vi "Port.vi"(8 "error in (no error)":errorcluster, 11 "Node Ptr":T2 format="%.0x") -> (0 "error out":errorcluster)   [LabVIEW 2020, in "Communication Bus Template System Explorer.lvlib" / "Implementation.lvlib"]
uses:
  Implementation.lvlib
  <vilib>/NI VeriStand/Custom Device API/Custom Device Item Ref.ctl
  Types/XNET Interface Name.ctl
  <vilib>/NI VeriStand/Custom Device API/Custom Device API.lvlib
  Scripting/Communication Bus Template Scripting.lvlib
panel:
  out "CAN Cluster":string
  in  "XNET Interface Name":T1
  in  "Baud Rate":u32
  in  "Database":string(combo)
  in  "SHDocVw.IWebBrowser":refnum<k7>(container)
  in  "Specific Header":cluster{"Section Name":string}={"Section Name"="Specific Page Settings"}
  in  "General Header":cluster{"Section Name":string}={"Section Name"="General Page Settings"}
  in  "Description":string
  in  "Name":string
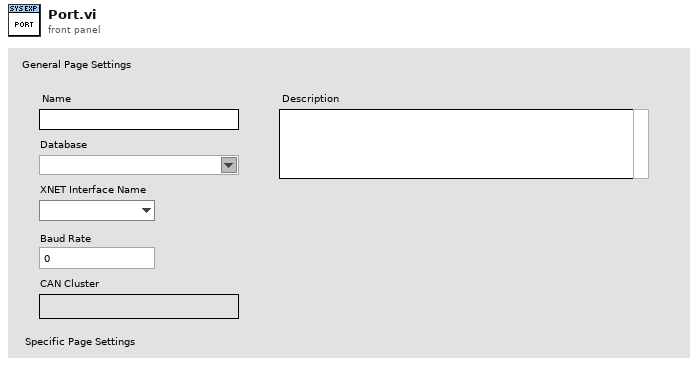
[diagram p1: front panel]
types:
  T1 = typedef "Communication Bus Template System Explorer.lvlib/Implementation.lvlib/XNET Interface Name.ctl" = u16
  T2 = typedef "Custom Device API.lvlib/Custom Device Item Ref.ctl" = u64
  T3 = typedef "Custom Device API.lvlib/Custom Device Item Info.ctl" = cluster{"Name":string, "Is Channel":bool, "GUID":string, "Is Waveform":bool}
  T4 = typedef "Custom Device API.lvlib/Custom Device Commands.ctl" = enum16{"Default", "Item renamed", "Shutdown", "Dynamic button pressed"}
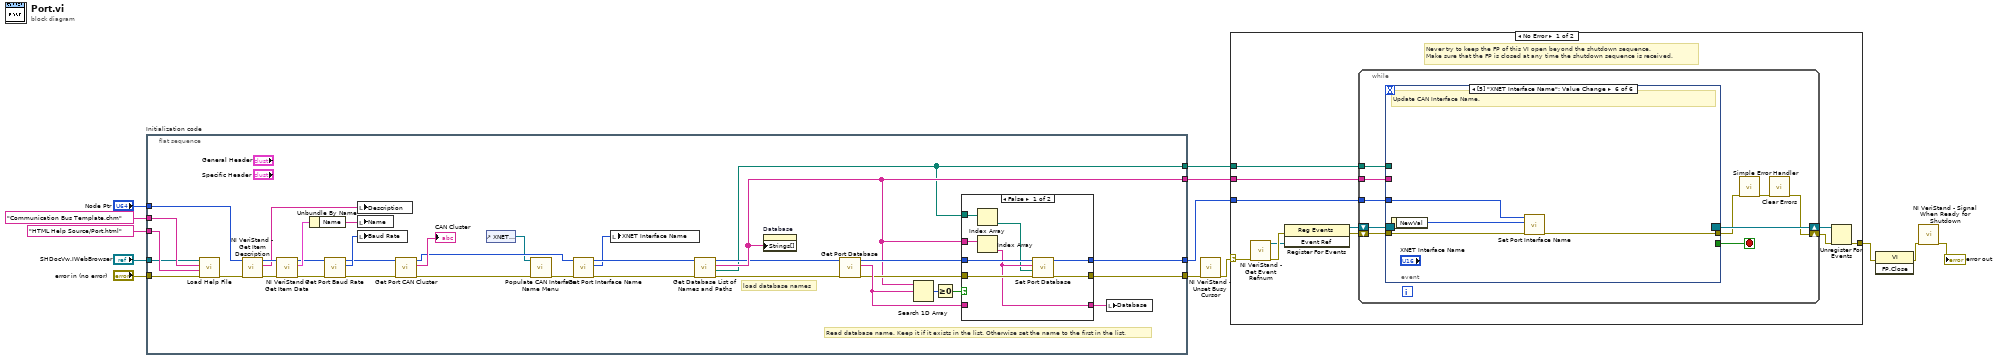
[diagram p0: block diagram]
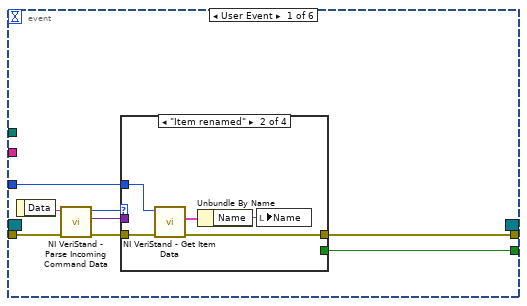
[diagram p3: hidden frame]
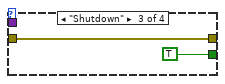
[diagram p5: hidden frame]
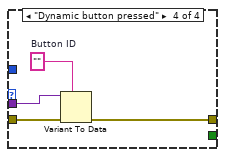
[diagram p6: hidden frame]
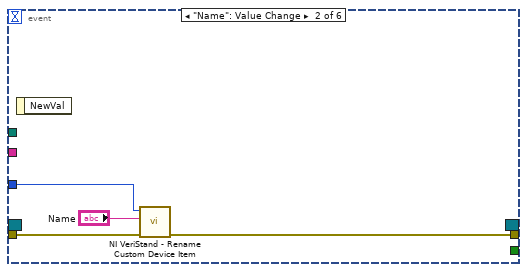
[diagram p7: hidden frame]
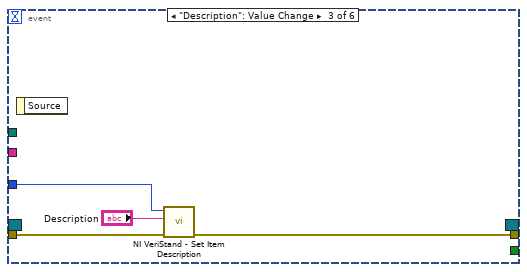
[diagram p8: hidden frame]
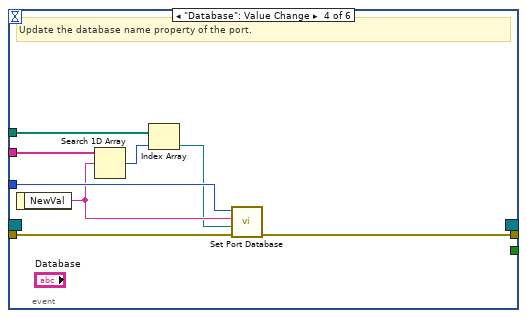
[diagram p9: hidden frame]
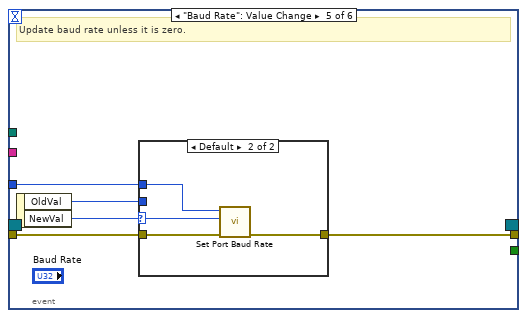
[diagram p10: hidden frame]
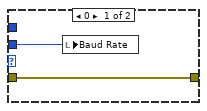
[diagram p11: hidden frame]
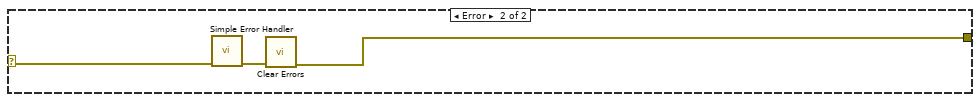
[diagram p12: hidden frame]
diagram:
  n1 = flat-sequence "Initialization code" {
    tunnel: "error in (no error)" -> [w43]
    tunnel: "Node Ptr" -> [w46]
    tunnel: [w23] -> w9
    tunnel: [w24] -> w6
    tunnel: "SHDocVw.IWebBrowser" -> [w39]
    tunnel: "HTML Help Source/Port.html" ("CD_CHM_Section") -> [w41]
    tunnel: "Communication Bus Template.chm" ("CD_CHM_FileName") -> [w40]
    tunnel: [w26] -> w2
    tunnel: [w30] -> w1
    frame #0 {
      # "Read database name. Keep it if it exists in the list. Otherwise set the name to the first in the list."
      # "load database names"
      n2 = call "Load Help File.vi"("error in (no error)"=w43, "HTML File to Load"=w41, "Main CHM File"=w40, "Browser"=w39) -> ("error out"=w42:errorcluster)  [unwired: 7 in]
      n3 = call <vilib>:"NI VeriStand - Get Item Description.vi"("error in (no error)"=w42, "Item Ref in"=w46) -> ("error out"=w48:errorcluster, "Description"=w44:string, "Item Ref out"=w49:T2)  [unwired: 7 out]
      n4 = call <vilib>:"NI VeriStand - Get Item Data.vi"("error in (no error)"=w48, "Item Ref in"=w49) -> ("error out"=w32:errorcluster, "Item Info"=w47:T3, "Item Ref out"=w31:T2)  [unwired: 7 out]
      n5 = Unbundle By Name(w47) -> ("Name"=w45:string)
      n6 = call "Get Port Baud Rate.vi"("error in"=w32, "Port Ref"=w31) -> ("error out"=w17:errorcluster, "Baud Rate"=w33:u32, "Port Ref out"=w18:T2)  [unwired: 7 in]
      n7 = local write "Description"(w44) -> ()
      n8 = local write "Name"(w45) -> ()
      n9 = local write "Baud Rate"(w33) -> ()
      n10 = call "Get Port CAN Cluster.vi"("error in"=w17, "Port Ref"=w18) -> ("error out"=w16:errorcluster, "CAN Cluster"=→"CAN Cluster":string, "Port Ref out"=w19:T2)  [unwired: 7 in]
      n11 = control-ref of="XNET Interface Name"() -> (w14:refnum<vi>)
      n12 = call "Populate CAN Interface Name Menu.vi"("error in"=w16, "CAN Interface Menu Refnum"=w14) -> ("error out"=w15:errorcluster)  [unwired: 9 in]
      n13 = call "Get Port Interface Name.vi"("error in"=w15, "Port Ref"=w19) -> ("error out"=w21:errorcluster, "CAN Interface Number"=w20:u16, "Port Ref out"=w22:T2)  [unwired: 6 in, 1 out]
      n14 = local write "XNET Interface Name"(w20) -> ()
      n15 = call "Get Database List of Names and Paths.vi"("error in"=w21, "Databases section Ref"=w22) -> ("error out"=w28:errorcluster, "Paths"=w26:path[], "Names"=w30:string[], "Databases section Ref out"=w29:T2)  [unwired: 6 in]
      n16 = property on="Database" class="CmbBox"("Strings[]"=w30) -> ()  [unwired: 2 in, 2 out]
      n17 = call "Get Port Database.vi"("error in"=w28, "Port Ref"=w29) -> ("error out"=w34:errorcluster, "Database Name"=w35:string, "Port Ref out"=w38:T2)  [unwired: 5 in, 2 out]
      n18 = Search 1D Array(1D array=w30, element=w35) -> (index of element=w27:i32)  [unwired: 1 in]
      n19 = Greater Or Equal To 0?(x=w27) -> (x >= 0?=w37:bool)
      n20 = case shown="False" w37 {
        tunnel: [w54 w59] -> w23
        tunnel: [w55 w60] -> w24
        tunnel: w34 -> [w53 w59]
        tunnel: w38 -> [w56 w60]
        tunnel: [w52 w58] -> w36
        tunnel: w35 -> [_ w58]
        tunnel: w30 -> [w57 _]
        tunnel: w26 -> [w51 _]
        frame False {
          n21 = Index Array(array=w51) -> (element=w50:path)  [unwired: 1 in]
          n22 = Index Array(array=w57) -> (element=w52:string)  [unwired: 1 in]
          n23 = call "Set Port Database.vi"("error in"=w53, "Database Path"=w50, "Database Name"=w52, "Port Ref"=w56) -> ("error out"=w54:errorcluster, "Port Ref out"=w55:T2)  [unwired: 6 in]
        }
        frame True {
        }
      }
      n24 = local write "Database"(w36) -> ()
    }
  }
  n25 = call <vilib>:"NI VeriStand - Unset Busy Cursor.vi"("error in (no error)"=w9) -> ("error out"=w8:errorcluster)  [unwired: 10 out]
  n26 = case shown="No Error" w8 {
    selector: w8 -> [w63 w135]
    tunnel: [w68 w133] -> w13
    tunnel: w6 -> [w64 _]
    tunnel: w2 -> [w62 _]
    tunnel: w1 -> [w61 _]
    frame No Error {
      # "Never try to keep the FP of this VI open beyond the shutdown sequence.\nMake sure that the FP is closed at any time the shutdown sequence is received."
      n27 = call <vilib>:"NI VeriStand - Get Event Refnum.vi"("error in (no error)"=w63) -> ("error out"=w71:errorcluster, "Event Ref"=w67:refnum<user-event>)  [unwired: 9 out]
      n28 = register-events(error in=w71, w67) -> (reference out=w65:refnum<event-registration>, error out=w66:errorcluster)  [unwired: 1 in]
      n29 = while {
        tunnel: w64 -> [w77]
        shift-right: [w74] -> w69
        shift-left: w66 -> [w80]
        shift-right: [w81] -> w70
        shift-left: w65 -> [w79]
        tunnel: w62 -> [w73]
        tunnel: w61 -> [w72]
        stop <- w78 stop-if-true
        n30 = event shown="[5] \"XNET Interface Name\": Value Change" {
          selector: w79 -> [_ _ _ _ _ _]
          dyn-events: [_ _ _ _ _ _] -> w81
          timeout: _ -> [_ _ _ _ _ _]
          tunnel: w80 -> [w89 w105 w108 w117 w122 w132]
          tunnel: [w85 _ _ _ _ _] -> w78
          tunnel: [w84 w104 w107 w113 w120 w130] -> w76
          tunnel: w77 -> [w83 w103 w109 w112 w119 w129]
          tunnel: w73 -> [_ _ _ w116 _ _]
          tunnel: w72 -> [_ _ _ w115 _ _]
          event User Event {
            n31 = event-data() -> ("Data"=w88:string)  [unwired: 1 out]
            n32 = call <vilib>:"NI VeriStand - Parse Incoming Command Data.vi"("error in (no error)"=w89, "Incoming data"=w88) -> ("error out"=w87:errorcluster, "Outgoing data"=w82:variant, "Action"=w86:T4)  [unwired: 7 out]
            n33 = case shown="\"Item renamed\"" w86 {
              tunnel: w87 -> [w90 w95 w96 w101]
              tunnel: [_ _ TRUE _] -> w85
              tunnel: [w90 w92 w96 w98] -> w84
              tunnel: w83 -> [_ w94 _ _]
              tunnel: w82 -> [_ _ _ w100]
              frame "Default", Default {
              }
              frame "Item renamed" {
                n34 = call <vilib>:"NI VeriStand - Get Item Data.vi"("error in (no error)"=w95, "Item Ref in"=w94) -> ("error out"=w92:errorcluster, "Item Info"=w93:T3)  [unwired: 8 out]
                n35 = Unbundle By Name(w93) -> ("Name"=w91:string)
                n36 = local write "Name"(w91) -> ()
              }
              frame "Shutdown" {
              }
              frame "Dynamic button pressed" {
                w99 = ""  # Button ID
                n37 = Variant To Data(error in=w101, type=w99, Variant=w100) -> (error out=w98:errorcluster)  [unwired: 1 out]
              }
            }
          }
          event "Name": Value Change {
            n38 = event-data() -> ()  [unwired: 2 out]
            n39 = call <vilib>:"NI VeriStand - Rename Custom Device Item.vi"("error in (no error)"=w105, "New Name"="Name", "Item Ref in"=w103) -> ("error out"=w104:errorcluster)  [unwired: 1 in, 7 out]
          }
          event "Description": Value Change {
            n40 = event-data() -> ()  [unwired: 2 out]
            n41 = call <vilib>:"NI VeriStand - Set Item Description.vi"("error in (no error)"=w108, "Description"="Description", "Item Ref in"=w109) -> ("error out"=w107:errorcluster)  [unwired: 8 out]
          }
          event "Database": Value Change {
            # "Update the database name property of the port."
            n42 = event-data() -> ("NewVal"=w111:string)  [unwired: 1 out]
            n43 = Search 1D Array(1D array=w115, element=w111) -> (index of element=w114:i32)  [unwired: 1 in]
            n44 = Index Array(array=w116, index=w114) -> (element=w110:path)
            n45 = call "Set Port Database.vi"("error in"=w117, "Database Path"=w110, "Database Name"=w111, "Port Ref"=w112) -> ("error out"=w113:errorcluster)  [unwired: 6 in, 1 out]
          }
          event "Baud Rate": Value Change {
            # "Update baud rate unless it is zero."
            n46 = event-data() -> ("OldVal"=w118:u32, "NewVal"=w121:u32)  [unwired: 1 out]
            n47 = case shown="Default" w121 {
              selector: w121 -> [_ w125]
              tunnel: w122 -> [w124 w128]
              tunnel: [w124 w127] -> w120
              tunnel: w119 -> [_ w126]
              tunnel: w118 -> [w123 _]
              frame 0 {
                n48 = local write "Baud Rate"(w123) -> ()
              }
              frame Default {
                n49 = call "Set Port Baud Rate.vi"("error in"=w128, "Baud Rate"=w125, "Port Ref"=w126) -> ("error out"=w127:errorcluster)  [unwired: 7 in, 1 out]
              }
            }
          }
          event Value Change {
            # "Update CAN Interface Name."
            n50 = event-data() -> ("NewVal"=w131:T1)  [unwired: 1 out]
            n51 = call "Set Port Interface Name.vi"("error in"=w132, "CAN Interface Number"=w131, "Port Ref"=w129) -> ("error out"=w130:errorcluster)  [unwired: 7 in, 1 out]
          }
        }
        n52 = call <vilib>:"Simple Error Handler.vi"("error in (no error)"=w76) -> ("error out"=w75:errorcluster)  [unwired: 1 in, 7 out]
        n53 = call <vilib>:"Clear Errors.vi"("error in (no error)"=w75) -> ("error out"=w74:errorcluster)  [unwired: 1 in, 5 out]
      }
      n54 = Unregister For Events(event registration refnum=w70, error in=w69) -> (error out=w68:errorcluster)
    }
    frame Error {
      n55 = call <vilib>:"Simple Error Handler.vi"("error in (no error)"=w135) -> ("error out"=w134:errorcluster)  [unwired: 1 in, 7 out]
      n56 = call <vilib>:"Clear Errors.vi"("error in (no error)"=w134) -> ("error out"=w133:errorcluster)  [unwired: 1 in, 5 out]
    }
  }
  n57 = invoke class="VI" method="FP.Close"(error in=w13) -> (error out=w12:errorcluster)  [unwired: 2 in, 2 out]
  n58 = call <vilib>:"NI VeriStand - Signal When Ready for Shutdown.vi"("error in (no error)"=w12) -> ("error out"=→"error out":errorcluster)  [unwired: 10 out]
